vi "SP - Get current VI name.vi"(8 "error in (no error)":errorcluster, 11 "JSON string":string) -> (0 "error out":errorcluster, 3 "value":string)   [LabVIEW 2020, in "ui-testing.lvlib"]
doc: "copyright: Thomas Zilliox©"
uses:
  ui-testing.lvlib
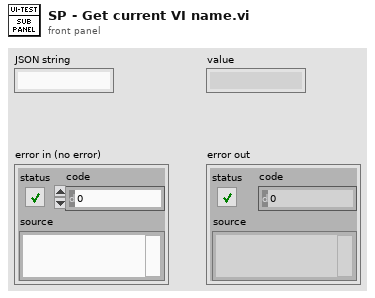
[diagram p1: front panel]
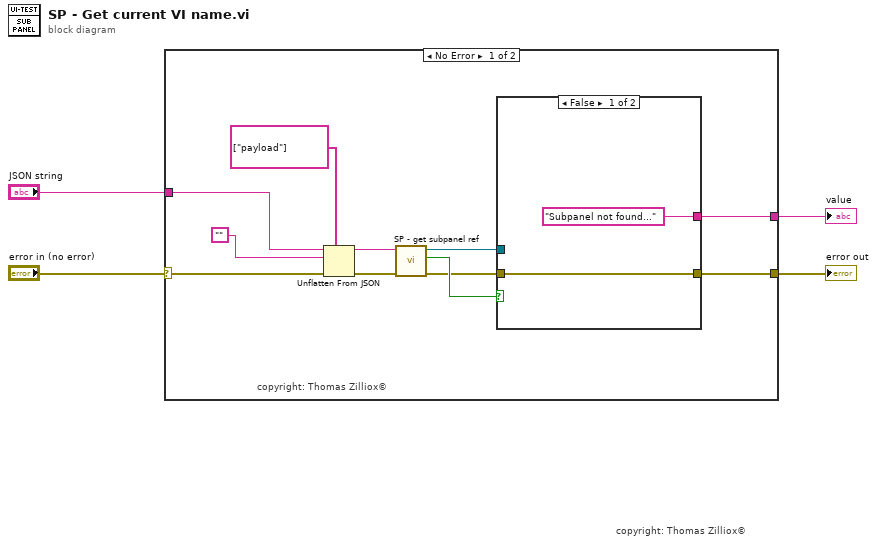
[diagram p0: block diagram]
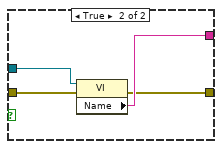
[diagram p2: hidden frame]
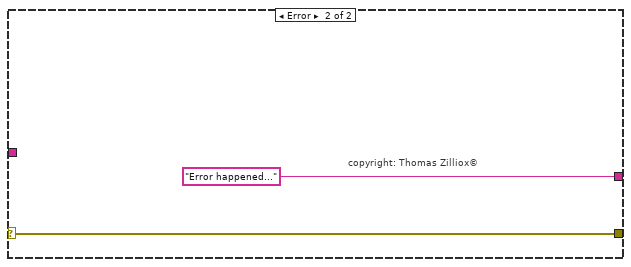
[diagram p3: hidden frame]
diagram:
  # "copyright: Thomas Zilliox©"
  n1 = case shown="No Error" "error in (no error)" {
    selector: "error in (no error)" -> [w11 w23]
    tunnel: "JSON string" -> [w12 _]
    tunnel: [w10 w23] -> w3
    tunnel: [w9 "Error happened..."] -> w1
    frame No Error {
      # "copyright: Thomas Zilliox©"
      n2 = Unflatten From JSON(path=string[] ["payload"], JSON string=w12, type and defaults="", error in (no error)=w11) -> (value=w8:string, error out=w14:errorcluster)  [unwired: 3 in]
      n3 = call "SP - get subpanel ref.vi"("error in (no error)"=w14, "subpanel"=w8) -> ("error out"=w5:errorcluster, "subpanel found ?"=w7:bool, "subpanel VI ref"=w6:refnum<vi>)  [unwired: 6 in, 1 out]
      n4 = case shown="False" w7 {
        tunnel: w5 -> [w16 w21]
        tunnel: [w16 w19] -> w10
        tunnel: ["Subpanel not found..." ("Name") w20] -> w9
        tunnel: w6 -> [_ w18]
        frame False {
        }
        frame True {
          n5 = property class="VI"(reference=w18, error in=w21) -> (error out=w19:errorcluster, "Name"=w20:string)  [unwired: 1 out]
        }
      }
    }
    frame Error {
      # "copyright: Thomas Zilliox©"
    }
  }
  "error out" <- w3
  "value" <- w1
